vi "Emergency Stop.vi"(8 "error in (no error)":errorcluster, 10 "Message In":refnum<class "Message.lvclass">, 11 "Root Actor in":refnum<class "Root Actor.lvclass">) -> (0 "error out":errorcluster, 3 "Root Actor out":refnum<class "Root Actor.lvclass">)   [LabVIEW 2024, in "Root Actor.lvclass"]
uses:
  Root Actor.lvclass
  Message/Message.lvclass
  Root Actor.lvclass/Root Actor.ctl
  Notifier Controller/Notifier Controller.lvclass
  Messenger/Messenger/Messenger.lvclass
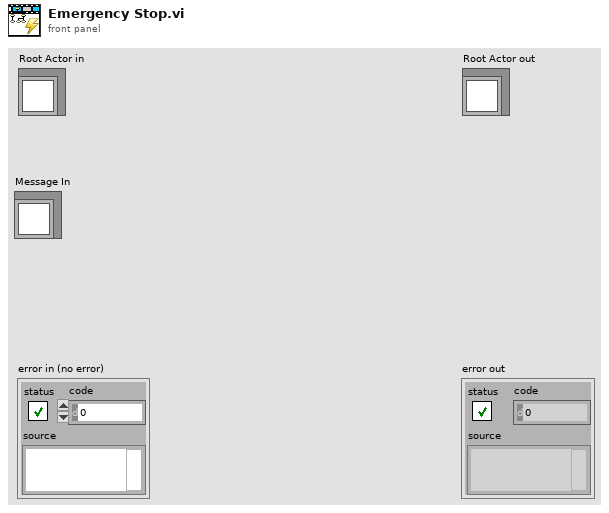
[diagram p1: front panel]
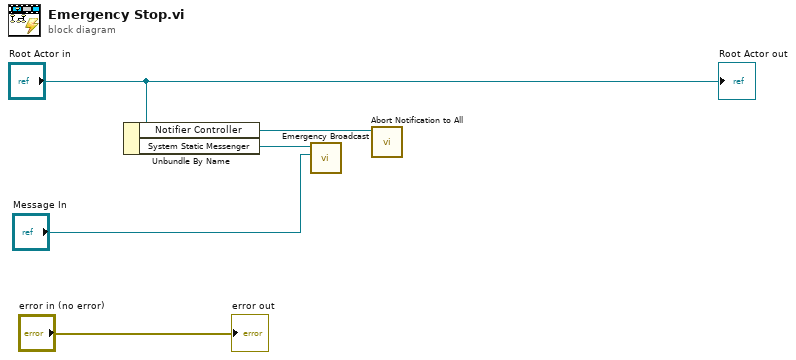
[diagram p0: block diagram]
diagram:
  n1 = Unbundle By Name("Root Actor in") -> ("Notifier Controller"=w1:refnum<class "Notifier Controller.lvclass">, "System Static Messenger"=w3:refnum<class "Messenger.lvclass">)
  n2 = call-dynamic "Emergency Broadcast.vi"("Message In"="Message In", "Messenger in"=w3) -> ()  [unwired: 8 in, 2 out]
  n3 = call-dynamic "Abort Notification to All.vi"("Notifier Controller in"=w1) -> ()  [unwired: 9 in, 2 out]
  "error out" <- "error in (no error)"
  "Root Actor out" <- "Root Actor in"
